vi "Timing Kernel.vi"(8 "error in (no error)":errorcluster, 9 "Time Limit (sec)":dbl, 10 "Timing Cmd In":T3, 11 "Timing params in":T1) -> (0 "error out":errorcluster, 2 "Done?":bool, 3 "Timing params Out":T1)   [LabVIEW 2018, in "Timing.lvlib" / "Timing Action Engine.lvlib"]
uses:
  Timing Action Engine.lvlib
  TimingCmd Enum.ctl
  TickCount.ctl
  Timing Params.ctl
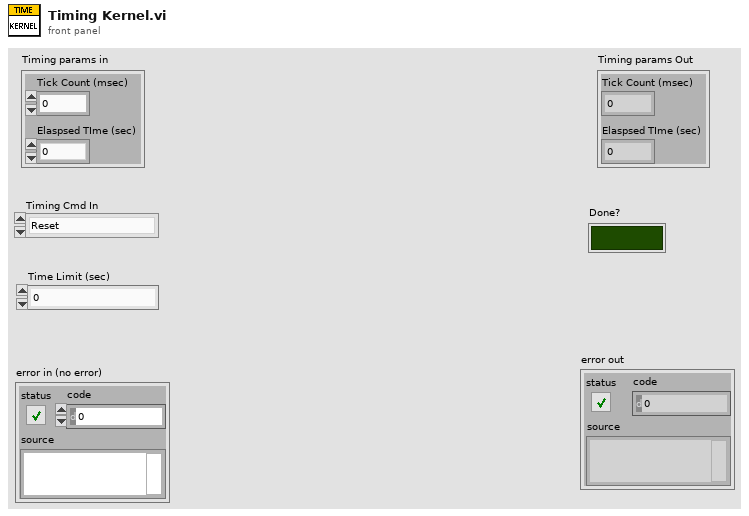
[diagram p1: front panel]
types:
  T1 = typedef "Timing.lvlib/Timing Action Engine.lvlib/Timing Params.ctl" = cluster{"Tick Count (msec)":T2, "Elaspsed TIme (sec)":dbl}
  T2 = typedef "Timing.lvlib/Timing Action Engine.lvlib/TickCount.ctl" = u32
  T3 = typedef "Timing.lvlib/Timing Action Engine.lvlib/TimingCmd Enum.ctl" = enum16{"Reset", "Pause", "Read Time"}
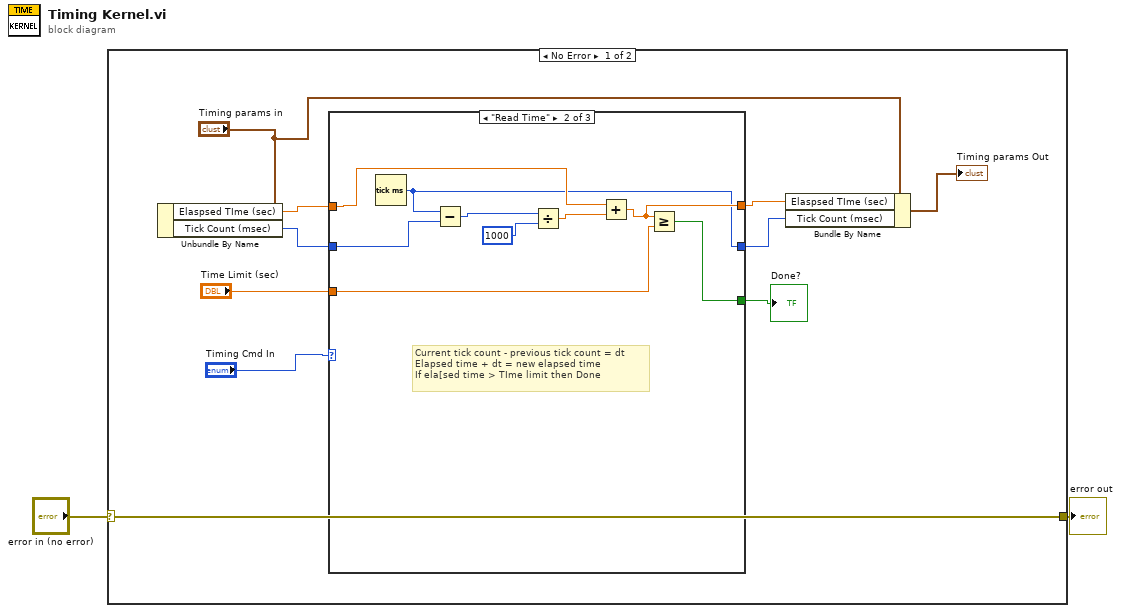
[diagram p0: block diagram]
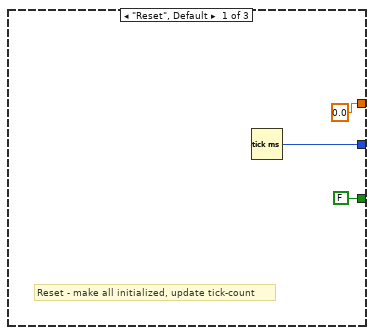
[diagram p2: hidden frame]
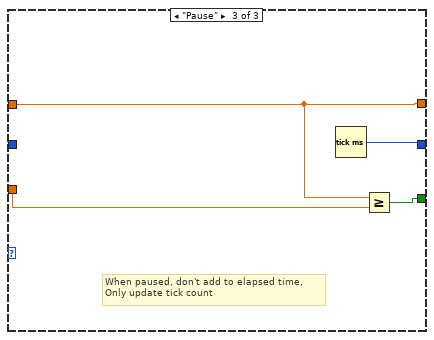
[diagram p3: hidden frame]
diagram:
  n1 = case shown="No Error" "error in (no error)" {
    selector: "error in (no error)" -> [w12 w29]
    tunnel: [w12 w29] -> w1
    frame No Error {
      n2 = Unbundle By Name("Timing params in") -> ("Elaspsed TIme (sec)"=w7:dbl, "Tick Count (msec)"=w8:T2)
      n3 = case shown="\"Read Time\"" "Timing Cmd In" {
        tunnel: w8 -> [_ w24 _]
        tunnel: [w14 w16 w25] -> w5
        tunnel: [0.0 w17 w26] -> w6
        tunnel: w7 -> [_ w20 w26]
        tunnel: "Time Limit (sec)" -> [_ w19 w27]
        tunnel: [FALSE w18 w28] -> w9
        frame "Reset", Default {
          # "Reset - make all initialized, update tick-count"
          n4 = Tick Count (ms)() -> (millisecond timer value=w14:u32)
        }
        frame "Read Time" {
          # "Current tick count - previous tick count = dt\nElapsed time + dt = new elapsed time\nIf ela[sed time > TIme limit then Done"
          n5 = Tick Count (ms)() -> (millisecond timer value=w16:u32)
          n6 = Subtract(x=w16, y=w24) -> (x-y=w23:T2)
          n7 = Divide(x=w23, y=u32 1000) -> (x/y=w21:dbl)
          n8 = Add(x=w20, y=w21) -> (x+y=w17:dbl)
          n9 = Greater Or Equal?(x=w17, y=w19) -> (x >= y?=w18:bool)
        }
        frame "Pause" {
          # "When paused, don't add to elapsed time, \nOnly update tick count"
          n10 = Tick Count (ms)() -> (millisecond timer value=w25:u32)
          n11 = Greater Or Equal?(x=w26, y=w27) -> (x >= y?=w28:bool)
        }
      }
      "Done?" <- w9
      n12 = Bundle By Name(cluster="Timing params in", "Elaspsed TIme (sec)"=w6, "Tick Count (msec)"=w5) -> (→"Timing params Out":T1)
    }
    frame Error {
    }
  }
  "error out" <- w1
